vi "Write Server Internal UEs.vi"(8 "error in (no error)":errorcluster, 10 "Server Internal UEs":T1, 11 "SignalGeneratorService in":refnum<class "NiDAQmx.lvclass">) -> (0 "error out":errorcluster, 3 "SignalGeneratorService out":refnum<class "NiDAQmx.lvclass">)   [LabVIEW 2021, in "NI DAQmx_server.lvlib" / "NiDAQmx.lvclass"]
uses:
  NiDAQmx.lvclass
  typeDefs/Server Internal UEs.ctl
  typeDefs/Server Internal Message.ctl
  NiDAQmx.lvclass/NiDAQmx.ctl
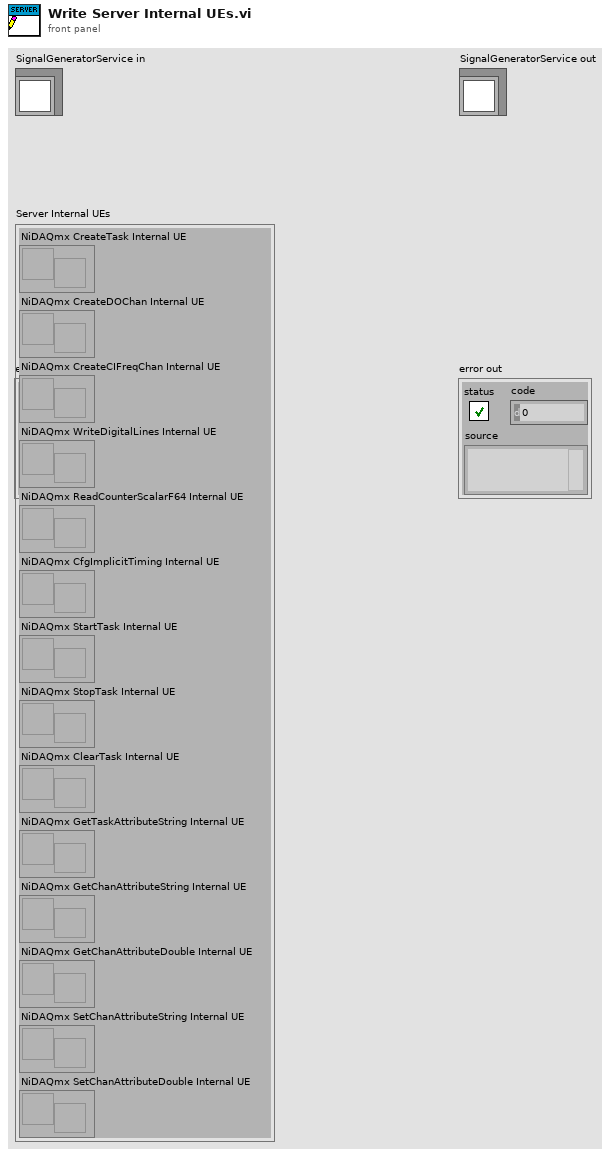
[diagram p1: front panel]
types:
  T1 = typedef "NI DAQmx_server.lvlib/NiDAQmx.lvclass/Server Internal UEs.ctl" = cluster{"NiDAQmx CreateTask Internal UE":refnum<user-event>, "NiDAQmx CreateDOChan Internal UE":refnum<user-event>, "NiDAQmx CreateCIFreqChan Internal UE":refnum<user-event>, "NiDAQmx WriteDigitalLines Internal UE":refnum<user-event>, "NiDAQmx ReadCounterScalarF64 Internal UE":refnum<user-event>, "NiDAQmx CfgImplicitTiming Internal UE":refnum<user-event>, "NiDAQmx StartTask Internal UE":refnum<user-event>, "NiDAQmx StopTask Internal UE":refnum<user-event>, "NiDAQmx ClearTask Internal UE":refnum<user-event>, "NiDAQmx GetTaskAttributeString Internal UE":refnum<user-event>, "NiDAQmx GetChanAttributeString Internal UE":refnum<user-event>, "NiDAQmx GetChanAttributeDouble Internal UE":refnum<user-event>, "NiDAQmx SetChanAttributeString Internal UE":refnum<user-event>, "NiDAQmx SetChanAttributeDouble Internal UE":refnum<user-event>}
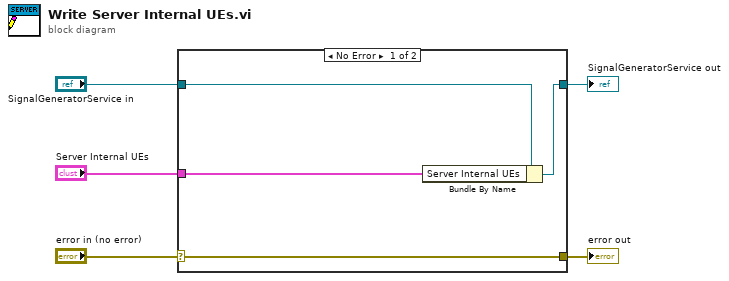
[diagram p0: block diagram]
diagram:
  n1 = case shown="No Error" "error in (no error)" {
    selector: "error in (no error)" -> [w9 w10]
    tunnel: [w9 w10] -> w4
    tunnel: [w7 w11] -> w2
    tunnel: "SignalGeneratorService in" -> [w8 w11]
    tunnel: "Server Internal UEs" -> [w6 _]
    frame No Error {
      n2 = Bundle By Name(cluster=w8, "Server Internal UEs"=w6) -> (w7:refnum<class "NiDAQmx.lvclass">)
    }
    frame Error {
    }
  }
  "error out" <- w4
  "SignalGeneratorService out" <- w2
